vi "GenerateStimulusOutputs_IOS_Optogenetics_test.vi"(0 "Trial duration (min)":dbl, 1 "Rest duration(s)":dbl, 2 "trial offset (s)":dbl, 3 "Left Pad":dbl, 4 "Right Pad":dbl, 5 "Auditory":dbl, 6 "LED":dbl, 8 "LED Stim Duration (s)":dbl, 9 "LED Stim Parameters":cluster{"Fs":dbl, "Samples":dbl}, 10 "LED Frequency":dbl, 11 "Sol Stim Parameters":cluster{"Fs":dbl, "Samples":dbl}, 12 "LED duty cycle (%)":dbl, 14 "Sol Stim Duration (s)":dbl, 16 "Sol Frequency":dbl, 18 "Sol Duty Cycle (%)":dbl) -> (13 "Double Left Puff":dbl[](array[numeric]), 15 "Double LED Out":dbl[](array[numeric]), 17 "Double Control Puff":dbl[](array[numeric]), 19 "Double Right Puff":dbl[](array[numeric]), 20 "Solenoid Stim Waveforms":digitalwaveform(graph), 22 "Stimulus Digital Outputs":digitalwaveform[](array[waveform]), 24 "Left Pad Out":digitalwaveform(graph), 25 "Auditory Out":digitalwaveform(graph), 26 "Right Pad Out":digitalwaveform(graph), 27 "LED Out":digitalwaveform(graph))   [LabVIEW 2018]
uses:
  <vilib>/Waveform/DWDTOps.llb/DWDT Analog to Digital.vi
  <vilib>/Waveform/DWDTOps.llb/DWDT Digital to Analog.vi
  <vilib>/measure/NI_MABase.lvlib
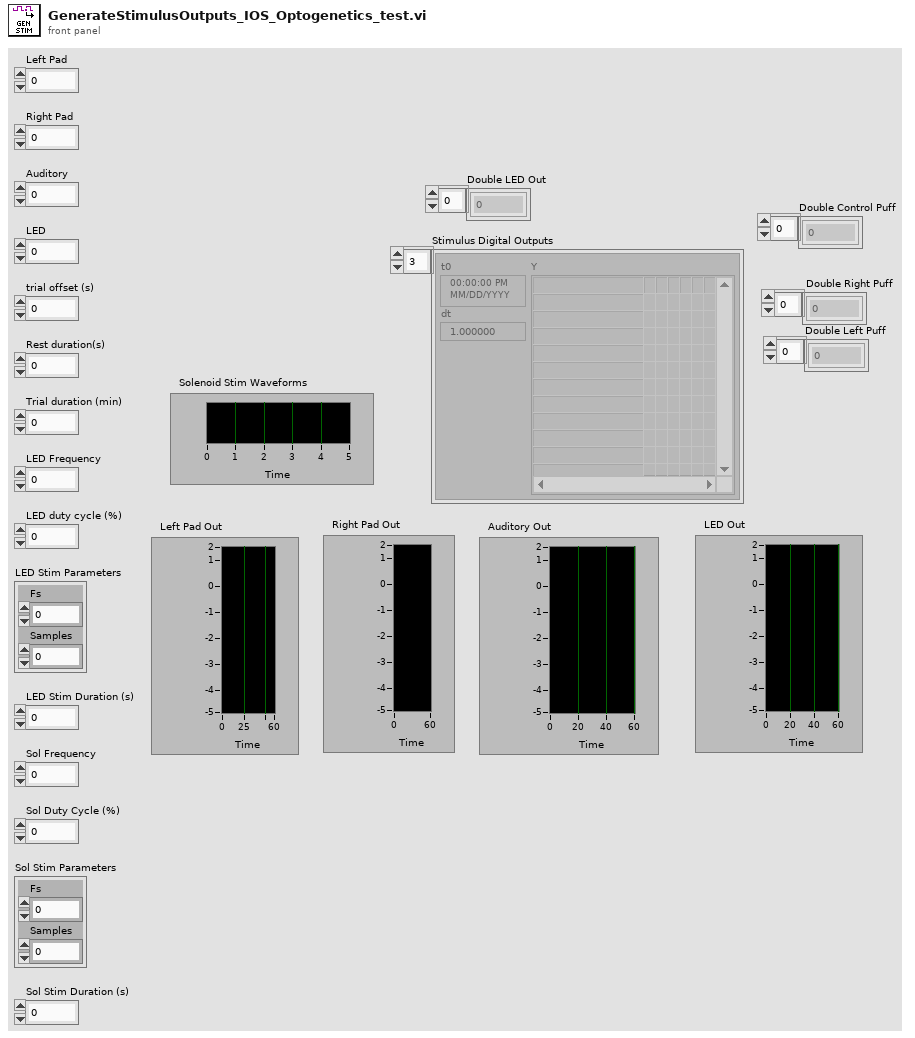
[diagram p1: front panel]
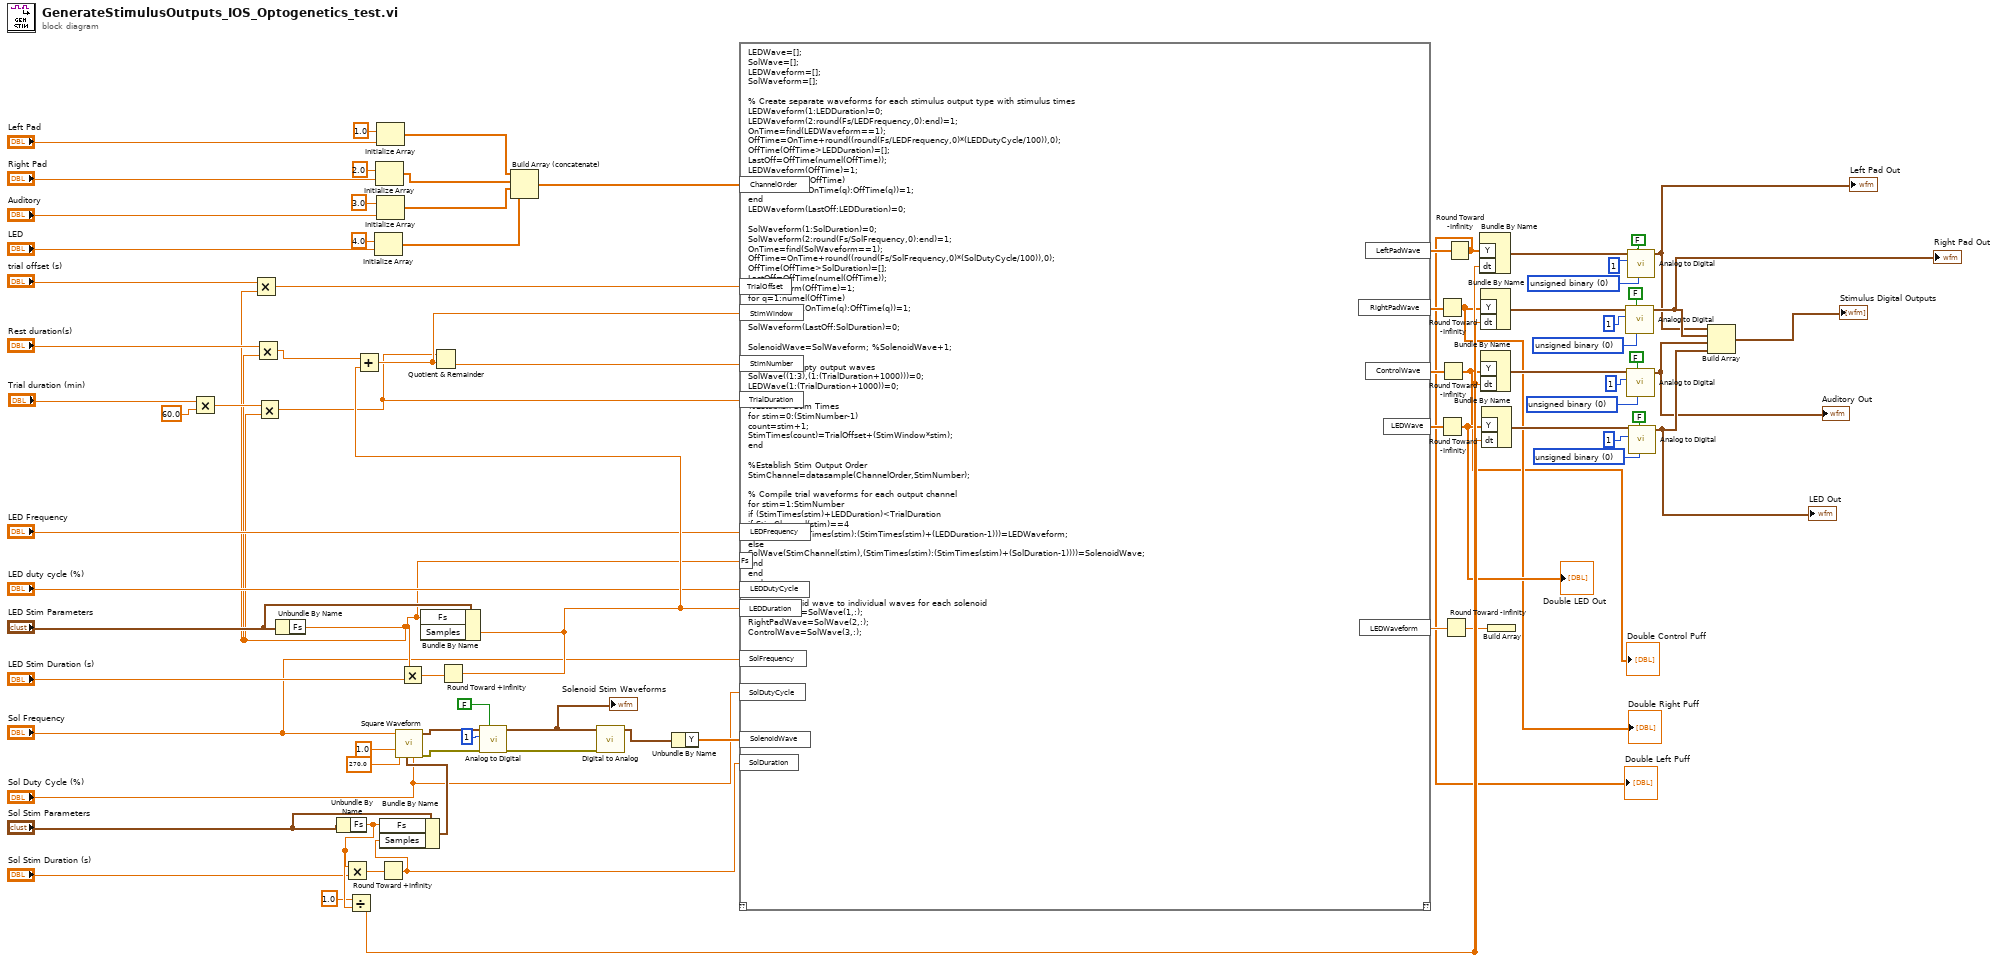
[diagram p0: block diagram]
diagram:
  w78 = u16 0 items=["unsigned binary", "offset binary", "2's complement"] ("data format (offset binary)")
  w77 = u16 0 items=["unsigned binary", "offset binary", "2's complement"] ("data format (offset binary)")
  w76 = u16 0 items=["unsigned binary", "offset binary", "2's complement"] ("data format (offset binary)")
  w75 = u16 0 items=["unsigned binary", "offset binary", "2's complement"] ("data format (offset binary)")
  n1 = Multiply(x="Trial duration (min)", y=60.0) -> (x*y=w21:dbl)
  n2 = Unbundle By Name("LED Stim Parameters") -> ("Fs"=w16:dbl)
  n3 = Multiply(x="trial offset (s)", y=w16) -> (x*y=w66:dbl)
  n4 = Multiply(x="Rest duration(s)", y=w16) -> (x*y=w25:dbl)
  n5 = Multiply(x=w21, y=w16) -> (x*y=w13:dbl)
  n6 = Unbundle By Name("Sol Stim Parameters") -> ("Fs"=w71:dbl)
  n7 = Multiply(x=w71, y="Sol Stim Duration (s)") -> (x*y=w53:dbl)
  n8 = Divide(x=1.0, y=w71) -> (x/y=w15:dbl)
  n9 = Initialize Array(4.0 ("element"), "LED") -> (w37:dbl[])
  n10 = Initialize Array(2.0 ("element"), "Right Pad") -> (w35:dbl[])
  n11 = Initialize Array(1.0 ("element"), "Left Pad") -> (w34:dbl[])
  n12 = Initialize Array(3.0 ("element"), "Auditory") -> (w36:dbl[])
  n13 = Round Toward +Infinity(x=w53) -> (ceil(x): smallest int >= x=w54:dbl)
  n14 = Bundle By Name(cluster="Sol Stim Parameters", "Fs"=w71, "Samples"=w54) -> (w41:cluster{"Fs":dbl, "Samples":dbl})
  n15 = call <vilib>:"Square Waveform.vi"("duty cycle (%)"="Sol Duty Cycle (%)", "sampling info"=w41, "phase"=270.0, "amplitude"=1.0, "frequency"="Sol Frequency") -> ("error out"=w44:errorcluster, "signal out"=w47:waveform(dbl))  [unwired: 5 in]
  n16 = Multiply(x=w16, y="LED Stim Duration (s)") -> (x*y=w52:dbl)
  n17 = Round Toward +Infinity(x=w52) -> (ceil(x): smallest int >= x=w80:dbl)
  n18 = Add(x=w25, y=w80) -> (x+y=w67:dbl)
  n19 = Bundle By Name(cluster="LED Stim Parameters", "Fs"=w16, "Samples"=w80) -> ()  [unwired: 1 out]
  n20 = Quotient & Remainder(x=w13, y=w67) -> (floor(x/y)=w64:dbl)  [unwired: 1 out]
  n21 = call-poly <vilib>:"Analog to Digital.vi"("compress digital (T)"=FALSE, "error in (no error)"=w44, "resolution (16 bit)"=1, "analog waveform"=w47) -> ("error out"=w45:errorcluster, "digital waveform"=w69:digitalwaveform)  [unwired: 4 in, 2 out]
  "Solenoid Stim Waveforms" <- w69
  n22 = Build Array (concatenate)(w34, w35, w36, w37) -> (w65:dbl[])
  n23 = call-poly <vilib>:"Digital to Analog.vi"("error in (no error)"=w45, "digital waveform"=w69) -> ("analog waveform"=w43:waveform(dbl))  [unwired: 6 in, 3 out]
  n24 = Unbundle By Name(w43) -> ("Y"=w63:dbl[])
  n25 = script code="LEDWave=[];\nSolWave=[];\nLEDWaveform=[];\nSolWaveform=[];\n\n% Create separate waveforms for each stimulus output type with stimulus times\nLEDWaveform(1:LEDDuration)=0;\nLEDWaveform(2:round(Fs/LEDFrequency,0):end)=1;\nOnTime=find(LEDWaveform==1);\nOffTime=OnTime+round((round(Fs/LEDFrequency,0)*(LEDDutyCycle/100)),0);\nOffTime(OffTime>LEDDuration)=[];\nLastOff=OffTime(numel(OffTime));\nLEDWaveform(OffTime)=1;\nfor q=1:numel(OffTime)\nLEDWaveform(OnTime(q):OffTime(q))=1;\nend\nLEDWaveform(LastOff:LEDDuration)=0;\n\nSolWaveform(1:SolDuration)=0;\nSolWaveform(2:round(Fs/SolFrequency,0):end)=1;\nOnTime=find(SolWaveform==1);\nOffTime=OnTime+round((round(Fs/SolFrequency,0)*(SolDutyCycle/100)),0);\nOffTime(OffTime>SolDuration)=[];\nLastOff=OffTime(numel(OffTime));\nSolWaveform(OffTime)=1;\nfor q=1:numel(OffTime)\nSolWaveform(OnTime(q):OffTime(q))=1;\nend\nSolWaveform(LastOff:SolDuration)=0;\n\nSolenoidWave=SolWaveform; %SolenoidWave+1;\n\n%initialize empty output waves\nSolWave((1:3),(1:(TrialDuration+1000)))=0;\nLEDWave(1:(TrialDuration+1000))=0;\n\n%Establish Stim Times\nfor stim=0:(StimNumber-1)\ncount=stim+1;\nStimTimes(count)=TrialOffset+(StimWindow*stim);\nend\n\n%Establish Stim Output Order\nStimChannel=datasample(ChannelOrder,StimNumber); \n\n% Compile trial waveforms for each output channel\nfor stim=1:StimNumber\nif (StimTimes(stim)+LEDDuration)<TrialDuration\nif StimChannel(stim)==4\nLEDWave(StimTimes(stim):(StimTimes(stim)+(LEDDuration-1)))=LEDWaveform;\nelse \nSolWave(StimChannel(stim),(StimTimes(stim):(StimTimes(stim)+(SolDuration-1))))=SolenoidWave;\nend\nend\nend\n\n%Split solenoid wave to individual waves for each solenoid\nLeftPadWave=SolWave(1,:);\nRightPadWave=SolWave(2,:);\nControlWave=SolWave(3,:);"("StimNumber"=w64, "ChannelOrder"=w65, "TrialDuration"=w13, "SolenoidWave"=w63, "LEDDuration"=w80, "SolDuration"=w54, "TrialOffset"=w66, "StimWindow"=w67, "LEDDutyCycle"="LED duty cycle (%)", "LEDFrequency"="LED Frequency", "Fs"=w16, "SolFrequency"="Sol Frequency", "SolDutyCycle"="Sol Duty Cycle (%)") -> ("LeftPadWave"=w81:dbl[], "RightPadWave"=w61:dbl[], "ControlWave"=w62:dbl[], "LEDWave"=w72:dbl[], "LEDWaveform"=w11:dbl)  [unwired: 1 in, 1 out]
  n26 = Round Toward -Infinity(1:w61) -> (0:w9:dbl[])
  "Double Right Puff" <- w9
  n27 = Round Toward -Infinity(1:w72) -> (0:w12:dbl[])
  "Double LED Out" <- w12
  n28 = Round Toward -Infinity(1:w62) -> (0:w7:dbl[])
  "Double Control Puff" <- w7
  n29 = Round Toward -Infinity(1:w11) -> (0:w10:dbl)
  n30 = Round Toward -Infinity(1:w81) -> (0:w8:dbl[])
  "Double Left Puff" <- w8
  n31 = Bundle By Name("Y"=w8, "dt"=w15) -> (w14:waveform(dbl))  [unwired: 1 in]
  n32 = Bundle By Name("Y"=w9, "dt"=w15) -> (w79:waveform(dbl))  [unwired: 1 in]
  n33 = Bundle By Name("Y"=w7, "dt"=w15) -> (w74:waveform(dbl))  [unwired: 1 in]
  n34 = Bundle By Name("Y"=w12, "dt"=w15) -> (w73:waveform(dbl))  [unwired: 1 in]
  n35 = Build Array(w10) -> ()  [unwired: 1 out]
  n36 = call-poly <vilib>:"Analog to Digital.vi"("data format (offset binary)"=w76, "compress digital (T)"=FALSE, "resolution (16 bit)"=1, "analog waveform"=w79) -> ("digital waveform"=w2:digitalwaveform)  [unwired: 4 in, 3 out]
  "Right Pad Out" <- w2
  n37 = call-poly <vilib>:"Analog to Digital.vi"("data format (offset binary)"=w77, "compress digital (T)"=FALSE, "resolution (16 bit)"=1, "analog waveform"=w74) -> ("digital waveform"=w3:digitalwaveform)  [unwired: 4 in, 3 out]
  "Auditory Out" <- w3
  n38 = call-poly <vilib>:"Analog to Digital.vi"("data format (offset binary)"=w75, "compress digital (T)"=FALSE, "resolution (16 bit)"=1, "analog waveform"=w14) -> ("digital waveform"=w1:digitalwaveform)  [unwired: 4 in, 3 out]
  "Left Pad Out" <- w1
  n39 = call-poly <vilib>:"Analog to Digital.vi"("data format (offset binary)"=w78, "compress digital (T)"=FALSE, "resolution (16 bit)"=1, "analog waveform"=w73) -> ("digital waveform"=w4:digitalwaveform)  [unwired: 4 in, 3 out]
  "LED Out" <- w4
  n40 = Build Array(w1, w2, w3, w4) -> (→"Stimulus Digital Outputs":digitalwaveform[])
